vi "Read Cooler Enqueuer.vi"(11 "冷却器控制器":refnum<class "Cooler Controller.lvclass">) -> (2 "冷却器待入队列":refnum<class "Message Enqueuer.lvclass">)   [LabVIEW 2013, in "Cooler Controller.lvlib" / "Cooler Controller.lvclass"]
doc: "该VI负责读取控制器正在控制的冷却器。由于控制器当前可能不负责控制任何冷却器，该VI可能返回“非法引用句柄”待入队列。"
uses:
  Cooler Controller.lvclass
  <vilib>/ActorFramework/Message Enqueuer/Message Enqueuer.lvclass
  Cooler Controller.lvclass/Cooler Controller.ctl
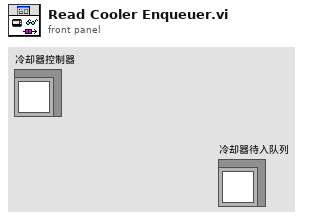
[diagram p1: front panel]
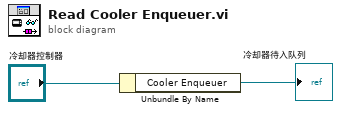
[diagram p0: block diagram]
diagram:
  n1 = Unbundle By Name("冷却器控制器") -> ("Cooler Enqueuer"=→"冷却器待入队列":refnum<class "Message Enqueuer.lvclass">)
